vi "Next RUN.vi"(8 "error in (no error)":errorcluster, 11 "Run Block in":refnum<class "Run Block.lvclass">) -> (0 "error out":errorcluster, 2 "Current RUN":refnum<class "Run Instance.lvclass">, 3 "Run Block out":refnum<class "Run Block.lvclass">)   [LabVIEW 2020, in "Run Utilities.lvlib" / "Run Block.lvclass"]
doc: "Move to next script in the schedule"
uses:
  Run Block.lvclass
  Run Instance/Run Instance.lvclass
  Run Block.lvclass/Run Block.ctl
  Schedule/Schedule.lvclass
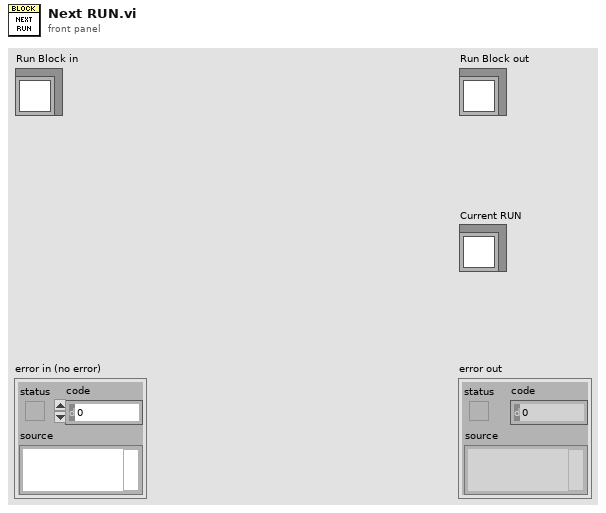
[diagram p1: front panel]
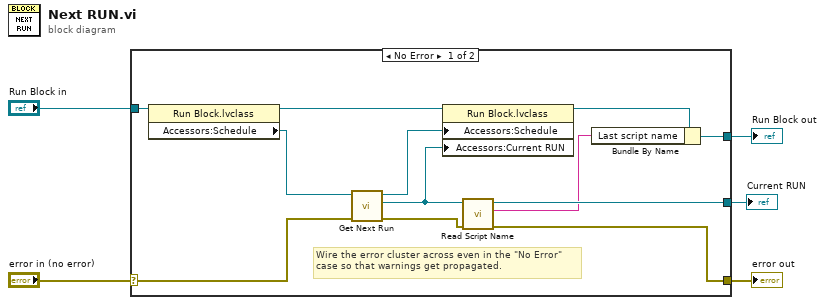
[diagram p0: block diagram]
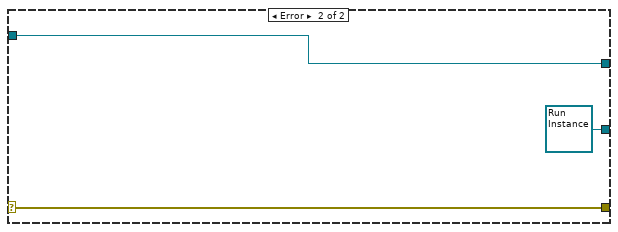
[diagram p2: hidden frame]
diagram:
  n1 = case shown="No Error" "error in (no error)" {
    selector: "error in (no error)" -> [w16 w20]
    tunnel: [w9 w20] -> w4
    tunnel: [w7 w19] -> w2
    tunnel: "Run Block in" -> [w17 w19]
    tunnel: [w11 refnum<class "Run Instance.lvclass"> refnum ("Run Instance")] -> w1
    frame No Error {
      # "Wire the error cluster across even in the \"No Error\"\ncase so that warnings get propagated."
      n2 = property class="Run Block.lvclass"(reference=w17) -> (reference out=w14:refnum<class "Run Block.lvclass">, "Accessors:Schedule"=w15:refnum<class "Schedule.lvclass">)  [unwired: 1 in, 1 out]
      n3 = call-dynamic "Get Next Run.vi"("error in (no error)"=w16, "Schedule in"=w15) -> ("error out"=w10:errorcluster, "Run Instance"=w12:refnum<class "Run Instance.lvclass">, "Schedule out"=w13:refnum<class "Schedule.lvclass">)  [unwired: 7 in]
      n4 = property class="Run Block.lvclass"(reference=w14, "Accessors:Schedule"=w13, "Accessors:Current RUN"=w12) -> (reference out=w8:refnum<class "Run Block.lvclass">)  [unwired: 1 in, 1 out]
      n5 = call-dynamic "Read Script Name.vi"("error in (no error)"=w10, "Run Instance in"=w12) -> ("error out"=w9:errorcluster, "Script Name"=w6:string, "Run Instance out"=w11:refnum<class "Run Instance.lvclass">)  [unwired: 7 in]
      n6 = Bundle By Name(cluster=w8, "Last script name"=w6) -> (w7:refnum<class "Run Block.lvclass">)
    }
    frame Error {
    }
  }
  "error out" <- w4
  "Run Block out" <- w2
  "Current RUN" <- w1
